vi "REPORT.Analog offset_.vi"(9 "Vasic":i32, 10 "Config Test IN":T1={"Config HW"={"VISA Rigol DP832"="USB0::0x1AB1::0x0E11::DP8C191500901::INSTR", "Config Rigol DP832"=[{"Channel"=0, "V Limit"=5.5, "I Limit"=0.5, "V Out"=5.0}, {"Channel"=1, "V Limit"=5.5, "I Limit"=0.8, "V Out"=5.0}, {"Channel"=2, "V Limit"=5.5, "I Limit"=0.2, "V Out"=0.0}], "CTA Test#"="CTA013 A", "FT_Handle"=432866568, "Espera acceso FT"=10, "VISA Tek MDO3104"="Rigol_DP832", "VISA Key 81160A"="Rigol_DP832"}, "Config Test"=[{"Vasic"=2.8, "Global Reset"=FALSE, "Test Register?"=FALSE, "Test ADC?"=FALSE, "Test ADC"={"Repeats ADC"=100, "Max Desviation"=0.1}, "Limits ADC"={"Low"=[1.9, 1.3, 0.65, 0.0, 1.6, 1.4, 1.4, 0.9, 2.1, 0.85, 1.9], "High"=[2.1, 1.5, 0.85, 0.1, 1.4, 1.2, 1.2, 0.7, 1.9, 0.65, 1.7]}, "Test Max PN Min NP?"=FALSE, "Limits Max PN Min NP"={"Max P Upper"=2.177000045776367, "Min P Upper"=1.474, "Max N Upper"=1.475, "Min N Upper"=0.818, "Max P Lower"=1.888, "Min P Lower "=1.321, "Max N Lower"=1.322, "Min N Lower"=0.73}, "Test Rate Scan?"=FALSE, "Vin Rate Scan"=[], "Limits Rate Scan"={"High"=[0.15, 0.242, 0.331, 0.425, 0.512, 0.6, 0.688, 0.774, 0.847, 0.91], "Low"=[0.021, 0.11, 0.189, 0.27, 0.347, 0.421, 0.487, 0.551, 0.601, 0.635]}, "Test Rate Scan Adders?"=FALSE, "Vin Rate Adders"=[], "Limits Rate Scan adders"={"High"=[], "Low"=[]}, "Test offset analog?"=FALSE, "Lim Offset Analog"={"Max Analog"=0.05, "Min Analog"=-0.05}, "Test offset digital?"=FALSE, "Lim offset Dig"={"Max Dig"=0.05}, "Vasic real f.a."=2.8, "IBIAS"=FALSE, "VALUE IBIAS"=63}, {"Vasic"=2.8, "Global Reset"=FALSE, "Test Register?"=FALSE, "Test ADC?"=FALSE, "Test ADC"={"Repeats ADC"=100, "Max Desviation"=0.1}, "Limits ADC"={"Low"=[1.9, 1.3, 0.65, 0.0, 1.6, 1.4, 1.4, 0.9, 2.1, 0.85, 1.9], "High"=[2.1, 1.5, 0.85, 0.1, 1.4, 1.2, 1.2, 0.7, 1.9, 0.65, 1.7]}, "Test Max PN Min NP?"=FALSE, "Limits Max PN Min NP"={"Max P Upper"=2.177000045776367, "Min P Upper"=1.474, "Max N Upper"=1.475, "Min N Upper"=0.818, "Max P Lower"=1.888, "Min P Lower "=1.321, "Max N Lower"=1.322, "Min N Lower"=0.73}, "Test Rate Scan?"=FALSE, "Vin Rate Scan"=[], "Limits Rate Scan"={"High"=[0.15, 0.242, 0.331, 0.425, 0.512, 0.6, 0.688, 0.774, 0.847, 0.91], "Low"=[0.021, 0.11, 0.189, 0.27, 0.347, 0.421, 0.487, 0.551, 0.601, 0.635]}, "Test Rate Scan Adders?"=FALSE, "Vin Rate Adders"=[], "Limits Rate Scan adders"={"High"=[], "Low"=[]}, "Test offset analog?"=FALSE, "Lim Offset Analog"={"Max Analog"=0.05, "Min Analog"=-0.05}, "Test offset digital?"=FALSE, "Lim offset Dig"={"Max Dig"=0.05}, "Vasic real f.a."=2.8, "IBIAS"=FALSE, "VALUE IBIAS"=63}, {"Vasic"=2.8, "Global Reset"=FALSE, "Test Register?"=FALSE, "Test ADC?"=FALSE, "Test ADC"={"Repeats ADC"=100, "Max Desviation"=0.1}, "Limits ADC"={"Low"=[1.9, 1.3, 0.65, 0.0, 1.6, 1.4, 1.4, 0.9, 2.1, 0.85, 1.9], "High"=[2.1, 1.5, 0.85, 0.1, 1.4, 1.2, 1.2, 0.7, 1.9, 0.65, 1.7]}, "Test Max PN Min NP?"=FALSE, "Limits Max PN Min NP"={"Max P Upper"=2.177000045776367, "Min P Upper"=1.474, "Max N Upper"=1.475, "Min N Upper"=0.818, "Max P Lower"=1.888, "Min P Lower "=1.321, "Max N Lower"=1.322, "Min N Lower"=0.73}, "Test Rate Scan?"=FALSE, "Vin Rate Scan"=[], "Limits Rate Scan"={"High"=[0.15, 0.242, 0.331, 0.425, 0.512, 0.6, 0.688, 0.774, 0.847, 0.91], "Low"=[0.021, 0.11, 0.189, 0.27, 0.347, 0.421, 0.487, 0.551, 0.601, 0.635]}, "Test Rate Scan Adders?"=FALSE, "Vin Rate Adders"=[], "Limits Rate Scan adders"={"High"=[], "Low"=[]}, "Test offset analog?"=FALSE, "Lim Offset Analog"={"Max Analog"=0.05, "Min Analog"=-0.05}, "Test offset digital?"=FALSE, "Lim offset Dig"={"Max Dig"=0.05}, "Vasic real f.a."=2.8, "IBIAS"=FALSE, "VALUE IBIAS"=63}, {"Vasic"=2.8, "Global Reset"=FALSE, "Test Register?"=FALSE, "Test ADC?"=FALSE, "Test ADC"={"Repeats ADC"=100, "Max Desviation"=0.1}, "Limits ADC"={"Low"=[1.9, 1.3, 0.65, 0.0, 1.6, 1.4, 1.4, 0.9, 2.1, 0.85, 1.9], "High"=[2.1, 1.5, 0.85, 0.1, 1.4, 1.2, 1.2, 0.7, 1.9, 0.65, 1.7]}, "Test Max PN Min NP?"=FALSE, "Limits Max PN Min NP"={"Max P Upper"=2.177000045776367, "Min P Upper"=1.474, "Max N Upper"=1.475, "Min N Upper"=0.818, "Max P Lower"=1.888, "Min P Lower "=1.321, "Max N Lower"=1.322, "Min N Lower"=0.73}, "Test Rate Scan?"=FALSE, "Vin Rate Scan"=[], "Limits Rate Scan"={"High"=[0.15, 0.242, 0.331, 0.425, 0.512, 0.6, 0.688, 0.774, 0.847, 0.91], "Low"=[0.021, 0.11, 0.189, 0.27, 0.347, 0.421, 0.487, 0.551, 0.601, 0.635]}, "Test Rate Scan Adders?"=FALSE, "Vin Rate Adders"=[], "Limits Rate Scan adders"={"High"=[], "Low"=[]}, "Test offset analog?"=FALSE, "Lim Offset Analog"={"Max Analog"=0.05, "Min Analog"=-0.05}, "Test offset digital?"=FALSE, "Lim offset Dig"={"Max Dig"=0.05}, "Vasic real f.a."=2.8, "IBIAS"=FALSE, "VALUE IBIAS"=63}], "Result"=[{"Vasic Volt"=0, "Test Registros"={"Default Register OK"=FALSE, "Pattern Default"=[], "Read Default"=[], "W/R Register OK"=FALSE, "Pattern W/R"=[], "Read W/R"=[]}, "Test Dacs"={"Desviacion OK"=FALSE, "Means"=[], "Deviations"=[], "Desviations OK"=[], "Means OK"=[], "Graph Histogram"=[]}, "Test Max-Min PN"={"Max P Mini N OK"=FALSE, "PTHT Max P Min N"=[], "PTHT Max P Min N OK"=[], "NTHT Max P Min N"=[], "NTHT Max P Min N OK"=[], "Min P Max N OK"=FALSE, "PTHT Max N Min P"=[], "PTHT Max N Min P OK"=[], "NTHT Max N Min P"=[], "NTHT Max N Min P OK"=[], "Ref"=[]}, "Test Rate Scan"={"Rate Scan OK"=FALSE, "DAC TH0,TH1,TH2"=[], "Volt HLTH"=[], "Rate HLTH OK"=[], "DAC TH3,TH4,TH5"=[], "Volt LLTH"=[], "Rate LLTH 2 OK"=[], "Scaler 0"=[], "Ref"=[], "OFFSET HLTH"=[], "OFFSET LLTH"=[], "Real Voltage"=[]}, "Test Rate Scan adders"={"Rate Scan Adders OK"=FALSE, "DAC TH0,TH1,TH2"=[], "Volt HLTH"=[], "Add HLTH OK"=[], "DAC TH3,TH4,TH5"=[], "Volt LLTH"=[], "Add LLTH 2 OK"=[], "Scaler 0"=[], "Ref"=[], "OFFSET HLTH"=[], "OFFSET LLTH"=[], "Real Voltage"=[]}, "Test Offset Analog"={"Offset Analog OK"=FALSE, "V ADDOUT"=[], "Offset OK"=[], "Ref"=[]}, "Test Offset Digital"={"Offset Digital OK"=FALSE, "SCALER 1 START"=[], "SCALER 1 STOP"=[], "THX START"=[], "THX STOP"=[], "VHLTH START"=[], "VHLTH STOP"=[], "Index 1 Start"=[], "index 1 Stop"=[], "SCALER 2 START"=[], "SCALER 2 STOP"=[], "THX+3 START"=[], "THX+3 STOP"=[], "VLLTH START"=[], "VLLTH STOP"=[], "Index 2 Start"=[], "index 2 Stop"=[], "Dig HLTH OK"=[], "Dig LLTH 2 OK"=[], "Ref"=[]}, "info hardware"={"Iout V1"=0.0, "Iout V2"=0.0, "Iout V3"=0.0, "Vout V1"=0.0, "Vout V2"=0.0, "Vout V3"=0.0, "Temp"=0.0}, "Test Offset Analog add"={"Offset Analog add OK"=FALSE, "V ADDOUT add"=[], "Offset add OK"=[], "Ref add"=[]}, "info temp"={"T Asic Registers"=0.0, "T Board Test. ADC"=0.0, "T Asic Max Min N P"=0.0, "T Adc count"=0.0, "T Asic Digital Offset"=0.0, "T Asic Analog Offset"=0.0, "T Asic Analog add"=0.0, "T Asic Rate Scan"=0.0, "T Asic Rate Scan Adders"=0.0, "T Final"=0.0}}, {"Vasic Volt"=0, "Test Registros"={"Default Register OK"=FALSE, "Pattern Default"=[], "Read Default"=[], "W/R Register OK"=FALSE, "Pattern W/R"=[], "Read W/R"=[]}, "Test Dacs"={"Desviacion OK"=FALSE, "Means"=[], "Deviations"=[], "Desviations OK"=[], "Means OK"=[], "Graph Histogram"=[]}, "Test Max-Min PN"={"Max P Mini N OK"=FALSE, "PTHT Max P Min N"=[], "PTHT Max P Min N OK"=[], "NTHT Max P Min N"=[], "NTHT Max P Min N OK"=[], "Min P Max N OK"=FALSE, "PTHT Max N Min P"=[], "PTHT Max N Min P OK"=[], "NTHT Max N Min P"=[], "NTHT Max N Min P OK"=[], "Ref"=[]}, "Test Rate Scan"={"Rate Scan OK"=FALSE, "DAC TH0,TH1,TH2"=[], "Volt HLTH"=[], "Rate HLTH OK"=[], "DAC TH3,TH4,TH5"=[], "Volt LLTH"=[], "Rate LLTH 2 OK"=[], "Scaler 0"=[], "Ref"=[], "OFFSET HLTH"=[], "OFFSET LLTH"=[], "Real Voltage"=[]}, "Test Rate Scan adders"={"Rate Scan Adders OK"=FALSE, "DAC TH0,TH1,TH2"=[], "Volt HLTH"=[], "Add HLTH OK"=[], "DAC TH3,TH4,TH5"=[], "Volt LLTH"=[], "Add LLTH 2 OK"=[], "Scaler 0"=[], "Ref"=[], "OFFSET HLTH"=[], "OFFSET LLTH"=[], "Real Voltage"=[]}, "Test Offset Analog"={"Offset Analog OK"=FALSE, "V ADDOUT"=[], "Offset OK"=[], "Ref"=[]}, "Test Offset Digital"={"Offset Digital OK"=FALSE, "SCALER 1 START"=[], "SCALER 1 STOP"=[], "THX START"=[], "THX STOP"=[], "VHLTH START"=[], "VHLTH STOP"=[], "Index 1 Start"=[], "index 1 Stop"=[], "SCALER 2 START"=[], "SCALER 2 STOP"=[], "THX+3 START"=[], "THX+3 STOP"=[], "VLLTH START"=[], "VLLTH STOP"=[], "Index 2 Start"=[], "index 2 Stop"=[], "Dig HLTH OK"=[], "Dig LLTH 2 OK"=[], "Ref"=[]}, "info hardware"={"Iout V1"=0.0, "Iout V2"=0.0, "Iout V3"=0.0, "Vout V1"=0.0, "Vout V2"=0.0, "Vout V3"=0.0, "Temp"=0.0}, "Test Offset Analog add"={"Offset Analog add OK"=FALSE, "V ADDOUT add"=[], "Offset add OK"=[], "Ref add"=[]}, "info temp"={"T Asic Registers"=0.0, "T Board Test. ADC"=0.0, "T Asic Max Min N P"=0.0, "T Adc count"=0.0, "T Asic Digital Offset"=0.0, "T Asic Analog Offset"=0.0, "T Asic Analog add"=0.0, "T Asic Rate Scan"=0.0, "T Asic Rate Scan Adders"=0.0, "T Final"=0.0}}, {"Vasic Volt"=0, "Test Registros"={"Default Register OK"=FALSE, "Pattern Default"=[], "Read Default"=[], "W/R Register OK"=FALSE, "Pattern W/R"=[], "Read W/R"=[]}, "Test Dacs"={"Desviacion OK"=FALSE, "Means"=[], "Deviations"=[], "Desviations OK"=[], "Means OK"=[], "Graph Histogram"=[]}, "Test Max-Min PN"={"Max P Mini N OK"=FALSE, "PTHT Max P Min N"=[], "PTHT Max P Min N OK"=[], "NTHT Max P Min N"=[], "NTHT Max P Min N OK"=[], "Min P Max N OK"=FALSE, "PTHT Max N Min P"=[], "PTHT Max N Min P OK"=[], "NTHT Max N Min P"=[], "NTHT Max N Min P OK"=[], "Ref"=[]}, "Test Rate Scan"={"Rate Scan OK"=FALSE, "DAC TH0,TH1,TH2"=[], "Volt HLTH"=[], "Rate HLTH OK"=[], "DAC TH3,TH4,TH5"=[], "Volt LLTH"=[], "Rate LLTH 2 OK"=[], "Scaler 0"=[], "Ref"=[], "OFFSET HLTH"=[], "OFFSET LLTH"=[], "Real Voltage"=[]}, "Test Rate Scan adders"={"Rate Scan Adders OK"=FALSE, "DAC TH0,TH1,TH2"=[], "Volt HLTH"=[], "Add HLTH OK"=[], "DAC TH3,TH4,TH5"=[], "Volt LLTH"=[], "Add LLTH 2 OK"=[], "Scaler 0"=[], "Ref"=[], "OFFSET HLTH"=[], "OFFSET LLTH"=[], "Real Voltage"=[]}, "Test Offset Analog"={"Offset Analog OK"=FALSE, "V ADDOUT"=[], "Offset OK"=[], "Ref"=[]}, "Test Offset Digital"={"Offset Digital OK"=FALSE, "SCALER 1 START"=[], "SCALER 1 STOP"=[], "THX START"=[], "THX STOP"=[], "VHLTH START"=[], "VHLTH STOP"=[], "Index 1 Start"=[], "index 1 Stop"=[], "SCALER 2 START"=[], "SCALER 2 STOP"=[], "THX+3 START"=[], "THX+3 STOP"=[], "VLLTH START"=[], "VLLTH STOP"=[], "Index 2 Start"=[], "index 2 Stop"=[], "Dig HLTH OK"=[], "Dig LLTH 2 OK"=[], "Ref"=[]}, "info hardware"={"Iout V1"=0.0, "Iout V2"=0.0, "Iout V3"=0.0, "Vout V1"=0.0, "Vout V2"=0.0, "Vout V3"=0.0, "Temp"=0.0}, "Test Offset Analog add"={"Offset Analog add OK"=FALSE, "V ADDOUT add"=[], "Offset add OK"=[], "Ref add"=[]}, "info temp"={"T Asic Registers"=0.0, "T Board Test. ADC"=0.0, "T Asic Max Min N P"=0.0, "T Adc count"=0.0, "T Asic Digital Offset"=0.0, "T Asic Analog Offset"=0.0, "T Asic Analog add"=0.0, "T Asic Rate Scan"=0.0, "T Asic Rate Scan Adders"=0.0, "T Final"=0.0}}, {"Vasic Volt"=0, "Test Registros"={"Default Register OK"=FALSE, "Pattern Default"=[], "Read Default"=[], "W/R Register OK"=FALSE, "Pattern W/R"=[], "Read W/R"=[]}, "Test Dacs"={"Desviacion OK"=FALSE, "Means"=[], "Deviations"=[], "Desviations OK"=[], "Means OK"=[], "Graph Histogram"=[]}, "Test Max-Min PN"={"Max P Mini N OK"=FALSE, "PTHT Max P Min N"=[], "PTHT Max P Min N OK"=[], "NTHT Max P Min N"=[], "NTHT Max P Min N OK"=[], "Min P Max N OK"=FALSE, "PTHT Max N Min P"=[], "PTHT Max N Min P OK"=[], "NTHT Max N Min P"=[], "NTHT Max N Min P OK"=[], "Ref"=[]}, "Test Rate Scan"={"Rate Scan OK"=FALSE, "DAC TH0,TH1,TH2"=[], "Volt HLTH"=[], "Rate HLTH OK"=[], "DAC TH3,TH4,TH5"=[], "Volt LLTH"=[], "Rate LLTH 2 OK"=[], "Scaler 0"=[], "Ref"=[], "OFFSET HLTH"=[], "OFFSET LLTH"=[], "Real Voltage"=[]}, "Test Rate Scan adders"={"Rate Scan Adders OK"=FALSE, "DAC TH0,TH1,TH2"=[], "Volt HLTH"=[], "Add HLTH OK"=[], "DAC TH3,TH4,TH5"=[], "Volt LLTH"=[], "Add LLTH 2 OK"=[], "Scaler 0"=[], "Ref"=[], "OFFSET HLTH"=[], "OFFSET LLTH"=[], "Real Voltage"=[]}, "Test Offset Analog"={"Offset Analog OK"=FALSE, "V ADDOUT"=[], "Offset OK"=[], "Ref"=[]}, "Test Offset Digital"={"Offset Digital OK"=FALSE, "SCALER 1 START"=[], "SCALER 1 STOP"=[], "THX START"=[], "THX STOP"=[], "VHLTH START"=[], "VHLTH STOP"=[], "Index 1 Start"=[], "index 1 Stop"=[], "SCALER 2 START"=[], "SCALER 2 STOP"=[], "THX+3 START"=[], "THX+3 STOP"=[], "VLLTH START"=[], "VLLTH STOP"=[], "Index 2 Start"=[], "index 2 Stop"=[], "Dig HLTH OK"=[], "Dig LLTH 2 OK"=[], "Ref"=[]}, "info hardware"={"Iout V1"=0.0, "Iout V2"=0.0, "Iout V3"=0.0, "Vout V1"=0.0, "Vout V2"=0.0, "Vout V3"=0.0, "Temp"=0.0}, "Test Offset Analog add"={"Offset Analog add OK"=FALSE, "V ADDOUT add"=[], "Offset add OK"=[], "Ref add"=[]}, "info temp"={"T Asic Registers"=0.0, "T Board Test. ADC"=0.0, "T Asic Max Min N P"=0.0, "T Adc count"=0.0, "T Asic Digital Offset"=0.0, "T Asic Analog Offset"=0.0, "T Asic Analog add"=0.0, "T Asic Rate Scan"=0.0, "T Asic Rate Scan Adders"=0.0, "T Final"=0.0}}], "Execucion Test"={"Vasic Actual"=0}, "Config VGA"={"Theoretical Voltage"=[0.1, 0.2, 0.3, 0.4, 0.5, 0.6, 0.7, 0.8, 0.9, 1.0], "Real Voltage"=[0.10285, 0.20714, 0.29957, 0.40485, 0.49571, 0.60685, 0.69771, 0.80114, 0.89714, 0.99885], "Pulse Width"=57344, "Frecuency Pulse"=1000000.0, "VGA Gain"=[9, 16, 24, 34, 43, 52, 61, 72, 81, 93]}, "Test Info"={"Asic"="", "Operator"="", "Place"="", "Time start"=timestamp(0 s since 1904-01-01), "Time stop"=timestamp(0 s since 1904-01-01)}, "Info machine"={"SO"="", "SO Name"="", "SO Ver"="", "SO Build"="", "CPU"="", "APP"="", "APP YEAR"="", "APP ver"="", "APP User"="", "APP Serail"="", "MAC"=[], "PC NAME"=[], "PC IP"=[], "BIOS MANU"="", "BIOS NAME"="", "BIOS SERIAL"="", "BOARD MANU"="", "BOARD NAME"="", "BOARD SERIAL"="", "Driver Version"="", "Library Version"="", "FPGA Ver"=0, "ID CTA board"=0, "LAST BOOT"="", "LABVIEW Ver"=0}, "Partial Report"="", "CONFIG GEN"=[]} {"CONFIG GEN"."Vasic Theorical" min=1.0 max=1000000.0 step=1.0 format="%#_6pV"; "CONFIG GEN"."Frequency" min=0.001 max=333000000.0 step=1000.0 format="%#_6pHz"; "CONFIG GEN"."Leading Edge Time" min=1e-09 max=1.0 step=1e-10 format="%#_6ps"; "CONFIG GEN"."Trailing Edge Time" min=1e-09 max=1.0 step=1e-10 format="%#_6ps"; "CONFIG GEN"."Delay" min=0.0 max=1.0 step=1e-12 format="%#_6ps"; "CONFIG GEN"."Trigger Level Sync" items=["ECL", "TTL"]; "CONFIG GEN"."Trigger Sync Out" items=["AB"=3, "B"=2, "A"=1, "None"=0]; "CONFIG GEN"."Load" min=1.0 max=1000000.0 step=1.0 format="%#_6p"; "CONFIG GEN"."DC Offset" min=-10.0 max=10.0 step=0.1 format="%#_6pV"; "CONFIG GEN"."Amplitude" min=0.05 max=5.0 step=0.001 format="%#_6pV"; "CONFIG GEN"."Width Time" min=1.5e-09 max=1.0 step=1e-10 format="%#_6ps"; "CONFIG GEN"."Channel" items=["Channel1"=1, "Channel2"=2]; "Config VGA"."Theoretical Voltage" format="%1.4f"; "Config VGA"."VGA Gain" format="%02x"; "Config VGA"."Frecuency Pulse" format="%0_2p"; "Config VGA"."Pulse Width" format="%04x"; "Config VGA"."Real Voltage" format="%1.5f"; "Config Test"."VALUE IBIAS" max=63 step=1; "Config Test"."Vasic real f.a." min=2.8 max=3.8 step=0.01 format="%.2g"; "Config Test"."Limits Rate Scan adders"."Low" format="%1.3f"; "Config Test"."Limits Rate Scan adders"."High" format="%1.3f"; "Config Test"."Limits ADC"."High" format="%1.4f"; "Config Test"."Limits ADC"."Low" format="%1.3f"; "Config Test"."Lim offset Dig"."Max Dig" format="%.3g"; "Config Test"."Lim Offset Analog"."Min Analog" format="%.3g"; "Config Test"."Lim Offset Analog"."Max Analog" format="%.3g"; "Config Test"."Limits Rate Scan"."Low" format="%1.4f"; "Config Test"."Limits Rate Scan"."High" format="%1.3f"; "Config Test"."Limits Max PN Min NP"."Min P Upper" format="%.3g"; "Config Test"."Limits Max PN Min NP"."Min P Lower" format="%.3g"; "Config Test"."Limits Max PN Min NP"."Max N Lower" format="%.3g"; "Config Test"."Limits Max PN Min NP"."Max N Upper" format="%.3g"; "Config Test"."Limits Max PN Min NP"."Min N Lower" format="%.3g"; "Config Test"."Limits Max PN Min NP"."Min N Upper" format="%.3g"; "Config Test"."Limits Max PN Min NP"."Max P Upper" format="%.3g"; "Config Test"."Limits Max PN Min NP"."Max P Lower" format="%.3g"; "Config Test"."Vasic" min=2.8 max=3.8 step=0.01 format="%.2g"; "Config HW"."Config Rigol DP832"."Channel" items=["+30V Channel 1", "+30V Channel 2", "+5V Channel 3"]; "Config HW"."Config Rigol DP832"."V Limit" format="%.1g"; "Config HW"."Config Rigol DP832"."I Limit" format="%.1g"; "Config HW"."Config Rigol DP832"."V Out" format="%.1g"; "Result"."Test Registros"."Read W/R" format="%04x"; "Result"."Test Registros"."Pattern W/R" format="%04x"; "Result"."Test Registros"."Read Default" format="%04x"; "Result"."Test Registros"."Pattern Default" format="%04x"}, 11 "Text In":string) -> (3 "Text Out":string)   [LabVIEW 2019]
uses:
  Test.ctl
  TEST.TEST CONFIG HW.ctl
  Rigol DP832/DP832_Control Channels.ctl
  TEST.TEST CONFIG TEST MATRIZ.ctl
  TEST.TEST CONFIG TEST.ctl
  TEST.TEST RESULT.ctl
  test_result fvasic.ctl
  TEST.TEST EXECUTION TEST.ctl
  TEST.TEST CONFIG VGA.ctl
  TEST.TEST TEST INFO.ctl
  TEST.TEST INFO PC.ctl
  GenPulse_configurar.ctl
panel:
  # "Modo 2\nModo 3\nModo 4\nModo 2\nModo 3\nModo 4"
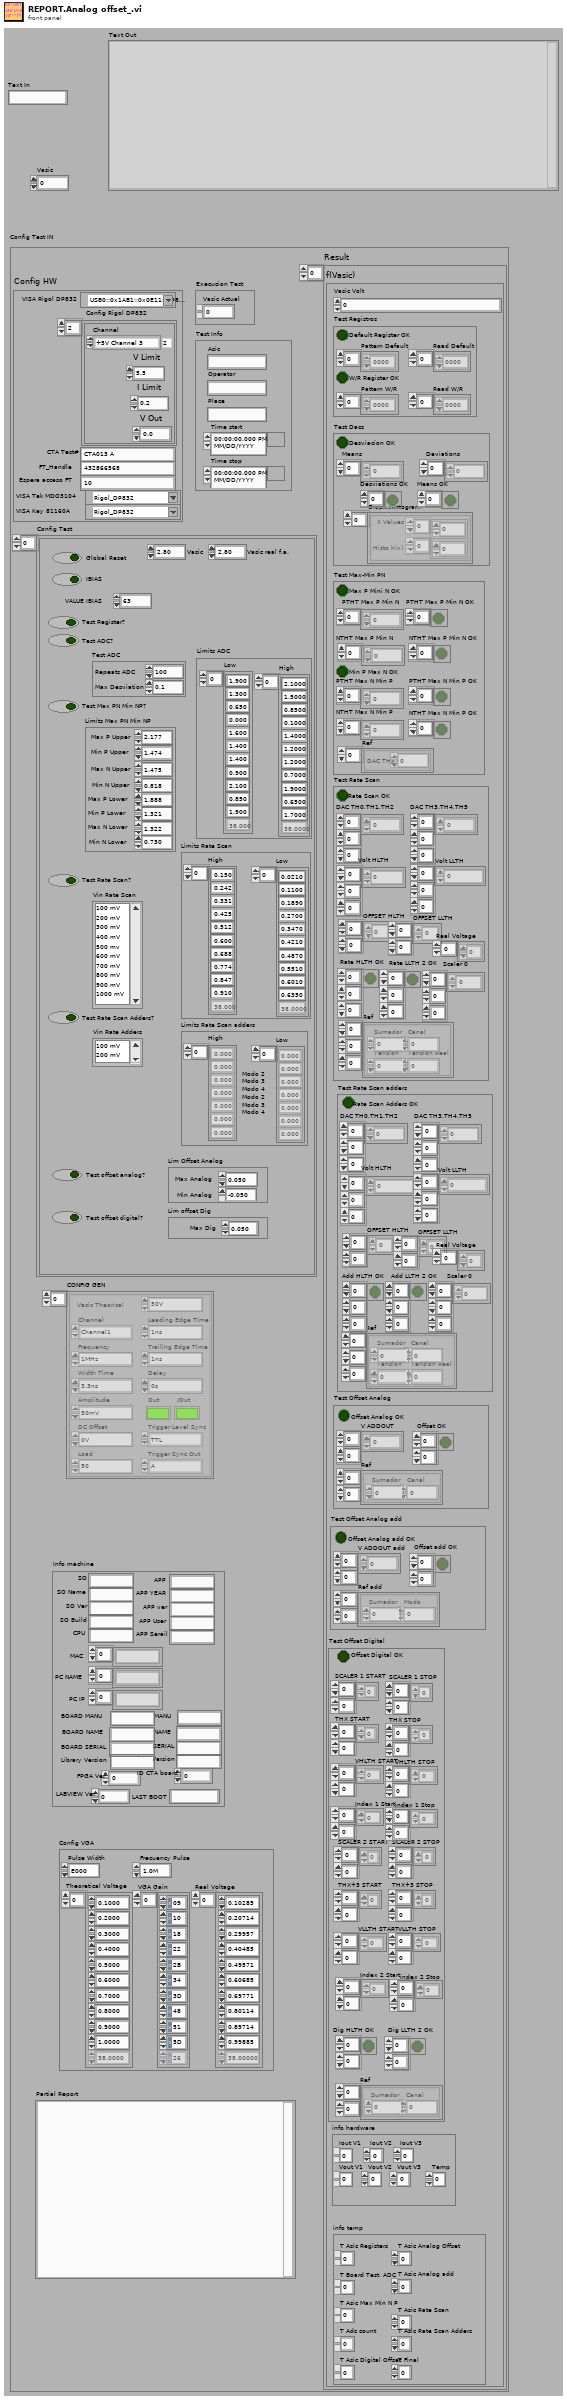
[diagram p1: front panel]
types:
  T1 = typedef "Test.ctl" = cluster{"Config HW":T2, "Config Test":T4, "Result":T6, "Execucion Test":T8, "Config VGA":T9, "Test Info":T10, "Info machine":T11, "Partial Report":string, "CONFIG GEN":T12[]}
  T2 = typedef "TEST.TEST CONFIG HW.ctl" = cluster{"VISA Rigol DP832":refnum<visa-resource-name>, "Config Rigol DP832":cluster{"Channel":T3, "V Limit":dbl, "I Limit":dbl, "V Out":dbl}[], "CTA Test#":string, "FT_Handle":u32, "Espera acceso FT":u32, "VISA Tek MDO3104":refnum<visa-resource-name>, "VISA Key 81160A":refnum<visa-resource-name>}
  T3 = typedef "DP832_Control Channels.ctl" = i32
  T4 = typedef "TEST.TEST CONFIG TEST MATRIZ.ctl" = T5[]
  T5 = typedef "TEST.TEST CONFIG TEST.ctl" = cluster{"Vasic":dbl, "Global Reset":bool, "Test Register?":bool, "Test ADC?":bool, "Test ADC":cluster{"Repeats ADC":i32, "Max Desviation":dbl}, "Limits ADC":cluster{"Low":dbl[], "High":dbl[]}, "Test Max PN Min NP?":bool, "Limits Max PN Min NP":cluster{"Max P Upper":dbl, "Min P Upper":dbl, "Max N Upper":dbl, "Min N Upper":dbl, "Max P Lower":dbl, "Min P Lower ":dbl, "Max N Lower":dbl, "Min N Lower":dbl}, "Test Rate Scan?":bool, "Vin Rate Scan":i32[], "Limits Rate Scan":cluster{"High":dbl[], "Low":dbl[]}, "Test Rate Scan Adders?":bool, "Vin Rate Adders":i32[], "Limits Rate Scan adders":cluster{"High":dbl[], "Low":dbl[]}, "Test offset analog?":bool, "Lim Offset Analog":cluster{"Max Analog":dbl, "Min Analog":dbl}, "Test offset digital?":bool, "Lim offset Dig":cluster{"Max Dig":dbl}, "Vasic real f.a.":dbl, "IBIAS":bool, "VALUE IBIAS":u8}
  T6 = typedef "TEST.TEST RESULT.ctl" = T7[]
  T7 = typedef "test_result fvasic.ctl" = cluster{"Vasic Volt":i32, "Test Registros":cluster{"Default Register OK":bool, "Pattern Default":u16[], "Read Default":u16[], "W/R Register OK":bool, "Pattern W/R":u16[], "Read W/R":u16[]}, "Test Dacs":cluster{"Desviacion OK":bool, "Means":dbl[], "Deviations":dbl[], "Desviations OK":bool[], "Means OK":bool[], "Graph Histogram":cluster{"X Values":dbl[], "Histo h(x)":i32[]}[]}, "Test Max-Min PN":cluster{"Max P Mini N OK":bool, "PTHT Max P Min N":dbl[], "PTHT Max P Min N OK":bool[], "NTHT Max P Min N":dbl[], "NTHT Max P Min N OK":bool[], "Min P Max N OK":bool, "PTHT Max N Min P":dbl[], "PTHT Max N Min P OK":bool[], "NTHT Max N Min P":dbl[], "NTHT Max N Min P OK":bool[], "Ref":cluster{"DAC THx":u8}[]}, "Test Rate Scan":cluster{"Rate Scan OK":bool, "DAC TH0,TH1,TH2":u16[][][], "Volt HLTH":dbl[][][], "Rate HLTH OK":bool[][][], "DAC TH3,TH4,TH5":u16[][][], "Volt LLTH":dbl[][][], "Rate LLTH 2 OK":bool[][][], "Scaler 0":u16[][][], "Ref":cluster{"Sumador":u8, "Canal":u8, "Tension":u8, "Tension Real":dbl}[][][], "OFFSET HLTH":dbl[][], "OFFSET LLTH":dbl[][], "Real Voltage":dbl[]}, "Test Rate Scan adders":cluster{"Rate Scan Adders OK":bool, "DAC TH0,TH1,TH2":u16[][][], "Volt HLTH":dbl[][][], "Add HLTH OK":bool[][][], "DAC TH3,TH4,TH5":u16[][][], "Volt LLTH":dbl[][][], "Add LLTH 2 OK":bool[][][], "Scaler 0":u16[][][], "Ref":cluster{"Sumador":u8, "Canal":u8, "Tension":u8, "Tension Real":dbl}[][][], "OFFSET HLTH":dbl[][], "OFFSET LLTH":dbl[][], "Real Voltage":dbl[]}, "Test Offset Analog":cluster{"Offset Analog OK":bool, "V ADDOUT":dbl[][], "Offset OK":bool[][], "Ref":cluster{"Sumador":u8, "Canal":u8}[][]}, "Test Offset Digital":cluster{"Offset Digital OK":bool, "SCALER 1 START":u16[][], "SCALER 1 STOP":u16[][], "THX START":u16[][], "THX STOP":u16[][], "VHLTH START":dbl[][], "VHLTH STOP":dbl[][], "Index 1 Start":i32[][], "index 1 Stop":i32[][], "SCALER 2 START":u16[][], "SCALER 2 STOP":u16[][], "THX+3 START":u16[][], "THX+3 STOP":u16[][], "VLLTH START":dbl[][], "VLLTH STOP":dbl[][], "Index 2 Start":i32[][], "index 2 Stop":i32[][], "Dig HLTH OK":bool[][], "Dig LLTH 2 OK":bool[][], "Ref":cluster{"Sumador":u8, "Canal":u8}[][]}, "info hardware":cluster{"Iout V1":dbl, "Iout V2":dbl, "Iout V3":dbl, "Vout V1":dbl, "Vout V2":dbl, "Vout V3":dbl, "Temp":dbl}, "Test Offset Analog add":cluster{"Offset Analog add OK":bool, "V ADDOUT add":dbl[][], "Offset add OK":bool[][], "Ref add":cluster{"Sumador":u8, "Modo":u8}[][]}, "info temp":cluster{"T Asic Registers":dbl, "T Board Test. ADC":dbl, "T Asic Max Min N P":dbl, "T Adc count":dbl, "T Asic Digital Offset":dbl, "T Asic Analog Offset":dbl, "T Asic Analog add":dbl, "T Asic Rate Scan":dbl, "T Asic Rate Scan Adders":dbl, "T Final":dbl}}
  T8 = typedef "TEST.TEST EXECUTION TEST.ctl" = cluster{"Vasic Actual":i32}
  T9 = typedef "TEST.TEST CONFIG VGA.ctl" = cluster{"Theoretical Voltage":dbl[], "Real Voltage":dbl[], "Pulse Width":u16, "Frecuency Pulse":dbl, "VGA Gain":u8[]}
  T10 = typedef "TEST.TEST TEST INFO.ctl" = cluster{"Asic":string, "Operator":string, "Place":string, "Time start":timestamp, "Time stop":timestamp}
  T11 = typedef "TEST.TEST INFO PC.ctl" = cluster{"SO":string, "SO Name":string, "SO Ver":string, "SO Build":string, "CPU":string, "APP":string, "APP YEAR":string, "APP ver":string, "APP User":string, "APP Serail":string, "MAC":string[], "PC NAME":string[], "PC IP":string[], "BIOS MANU":string, "BIOS NAME":string, "BIOS SERIAL":string, "BOARD MANU":string, "BOARD NAME":string, "BOARD SERIAL":string, "Driver Version":string, "Library Version":string, "FPGA Ver":u8, "ID CTA board":u64, "LAST BOOT":string, "LABVIEW Ver":u32}
  T12 = typedef "GenPulse_configurar.ctl" = cluster{"Channel":u16, "Frequency":dbl, "Width Time":dbl, "Amplitude":dbl, "DC Offset":dbl, "Load":dbl, "Leading Edge Time":dbl, "Trailing Edge Time":dbl, "Delay":dbl, "Out":bool, "/Out":bool, "Trigger Level Sync":u16, "Trigger Sync Out":u16, "Vasic Theorical":dbl}
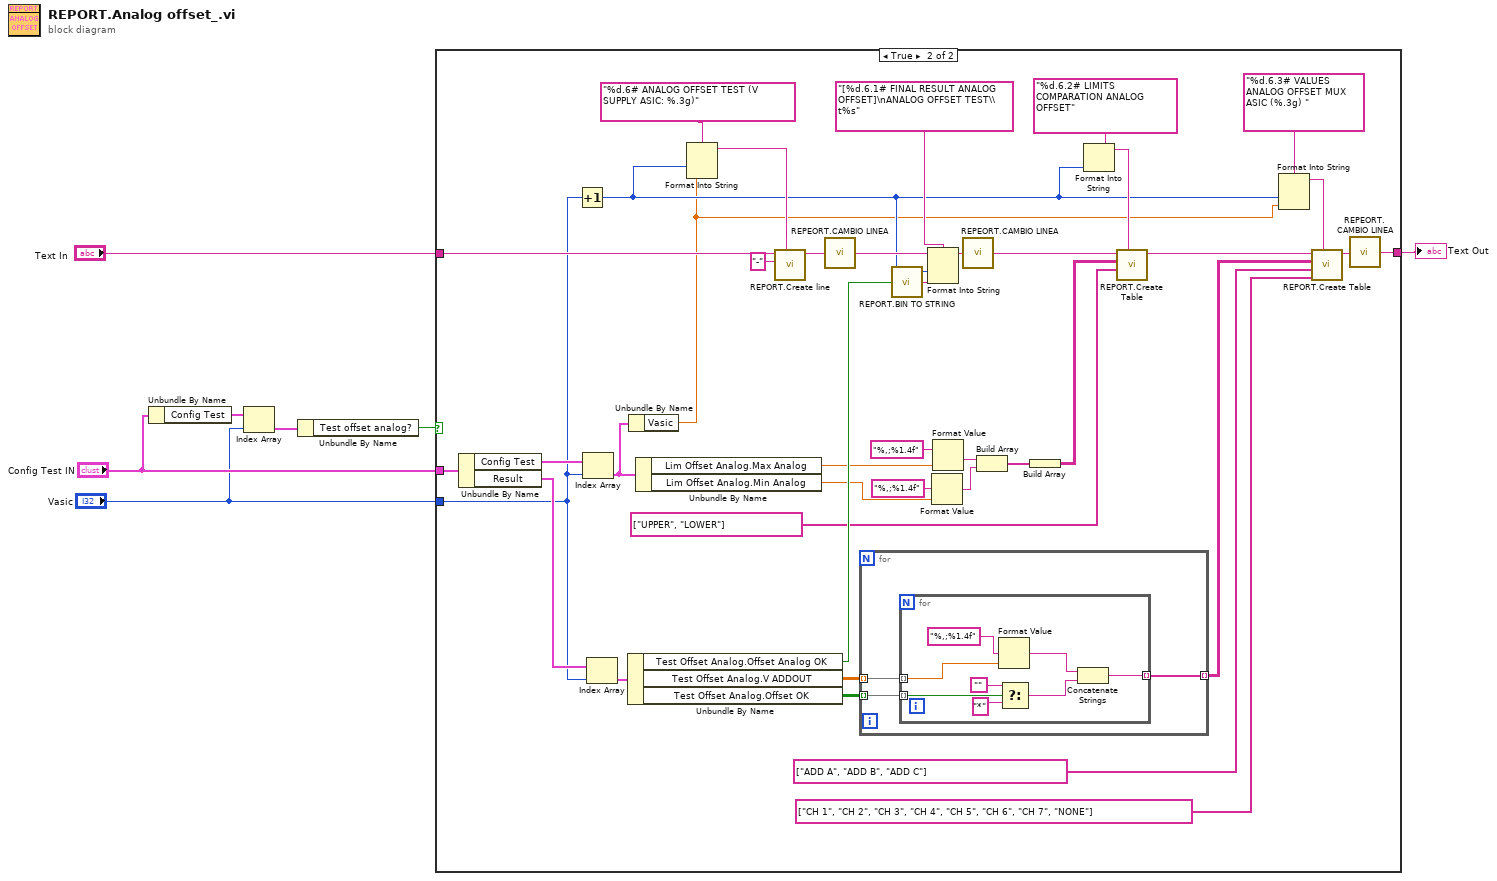
[diagram p0: block diagram]
diagram:
  n1 = Unbundle By Name("Config Test IN") -> ("Config Test"=w5:T4)
  n2 = Index Array(array=w5, index="Vasic") -> (element=w4:T5)
  n3 = Unbundle By Name(w4) -> ("Test offset analog?"=w1:bool)
  n4 = case shown="True" w1 {
    tunnel: "Text In" -> [w8 w48]
    tunnel: [w8 w44] -> w6
    tunnel: "Config Test IN" -> [_ w11]
    tunnel: "Vasic" -> [_ w10]
    frame False {
    }
    frame True {
      n5 = Unbundle By Name(w11) -> ("Config Test"=w43:T4, "Result"=w23:T6)
      n6 = Increment(x=w10) -> (x+1=w13:i32)
      n7 = Index Array(array=w43, index=w10) -> (element=w22:T5)
      n8 = Index Array(array=w23, index=w10) -> (element=w47:T7)
      n9 = Unbundle By Name(w47) -> ("Test Offset Analog.Offset Analog OK"=w42:bool, "Test Offset Analog.V ADDOUT"=w46:dbl[][], "Test Offset Analog.Offset OK"=w45:bool[][])
      n10 = Unbundle By Name(w22) -> ("Vasic"=w9:dbl)
      n11 = Unbundle By Name(w22) -> ("Lim Offset Analog.Max Analog"=w29:dbl, "Lim Offset Analog.Min Analog"=w28:dbl)
      n12 = Format Into String(format string="%d.6# ANALOG OFFSET TEST (V SUPPLY ASIC: %.3g)" ("Secction"), w13, w9) -> (resulting string=w20:string)  [unwired: 2 in, 1 out]
      n13 = call "REPORT.Create line.vi"("Secction"=w20, "Char"="-", "Text In"=w48) -> ("Text Out"=w25:string)  [unwired: 8 in]
      n14 = call "REPEORT.CAMBIO LINEA.vi"("Text Out"=w25) -> ("String"=w24:string)  [unwired: 8 in]
      n15 = for {
        tunnel: w46 -> [w51] mode=indexing
        tunnel: w45 -> [w49] mode=indexing
        tunnel: [w50] -> w26 mode=indexing
        n16 = for {
          tunnel: w51 -> [w59] mode=indexing
          tunnel: [w54] -> w50 mode=indexing
          tunnel: w49 -> [w53] mode=indexing
          n17 = Format Value(format string="%,;%1.4f", value (0)=w59) -> (output string=w52:string)  [unwired: 1 in]
          n18 = Select(t="", s=w53, f="*") -> (s? t:f=w55:string)
          n19 = Concatenate Strings(w52, w55) -> (w54:string)
        }
      }
      n20 = call "REPORT.BIN TO STRING.vi"("Resultado test"=w42) -> ("OK, Fault"=w18:string)  [unwired: 14 in]
      n21 = Format Into String(format string="[%d.6.1# FINAL RESULT ANALOG OFFSET]\nANALOG OFFSET TEST\\t%s" ("string"), initial string=w24, w13, w18) -> (resulting string=w40:string)  [unwired: 1 in, 1 out]
      n22 = Format Value(format string="%,;%1.4f", value (0)=w28) -> (output string=w34:string)  [unwired: 1 in]
      n23 = Format Value(format string="%,;%1.4f", value (0)=w29) -> (output string=w35:string)  [unwired: 1 in]
      n24 = call "REPEORT.CAMBIO LINEA.vi"("Text Out"=w40) -> ("String"=w17:string)  [unwired: 8 in]
      n25 = Build Array(w35, w34) -> (w33:string[])
      n26 = Build Array(w33) -> (w32:string[][])
      n27 = Format Into String(format string="%d.6.2# LIMITS COMPARATION ANALOG OFFSET" ("Secction"), w13) -> (resulting string=w15:string)  [unwired: 2 in, 1 out]
      n28 = call "REPORT.Create Table.vi"("Secction"=w15, "Column Headers"=string[] ["UPPER", "LOWER"], "Text 2d"=w32, "Text In"=w17) -> ("Text Out"=w27:string)  [unwired: 4 in, 1 out]
      n29 = Format Into String(format string="%d.6.3# VALUES ANALOG OFFSET MUX ASIC (%.3g) " ("Secction"), w13, w9) -> (resulting string=w12:string)  [unwired: 2 in, 1 out]
      n30 = call "REPORT.Create Table.vi"("Secction"=w12, "Row Headers"=string[] ["CH 1", "CH 2", "CH 3", "CH 4", "CH 5", "CH 6", "CH 7", "NONE"], "Column Headers"=string[] ["ADD A", "ADD B", "ADD C"], "Text 2d"=w26, "Text In"=w27) -> ("Text Out"=w30:string)  [unwired: 3 in, 1 out]
      n31 = call "REPEORT.CAMBIO LINEA.vi"("Text Out"=w30) -> ("String"=w44:string)  [unwired: 8 in]
    }
  }
  "Text Out" <- w6
